vi "FlexMag process file.vi"() -> ()   [LabVIEW 2018]
panel:
  in  "process name":string
  out "count":dbl
  out "multiple":string
  out "single":string
  in  "SEARCH":bool
  in  "EXIT":bool
  in  "SAVE":bool
  in  "DELETE":bool
  in  "ADD":bool
  # "Process Name"
  # "Recipe Name"
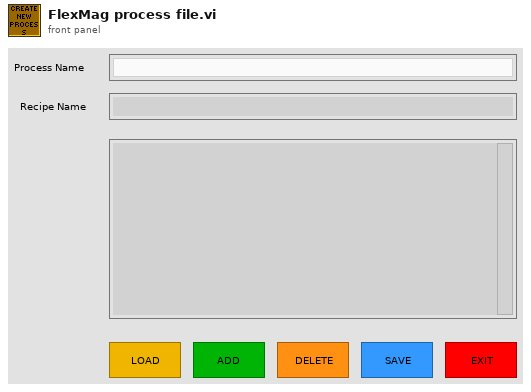
[diagram p1: front panel]
types:
  T1 = enum16{"open", "replace", "create", "open or create", "replace or create", "replace or create with confirmation"}
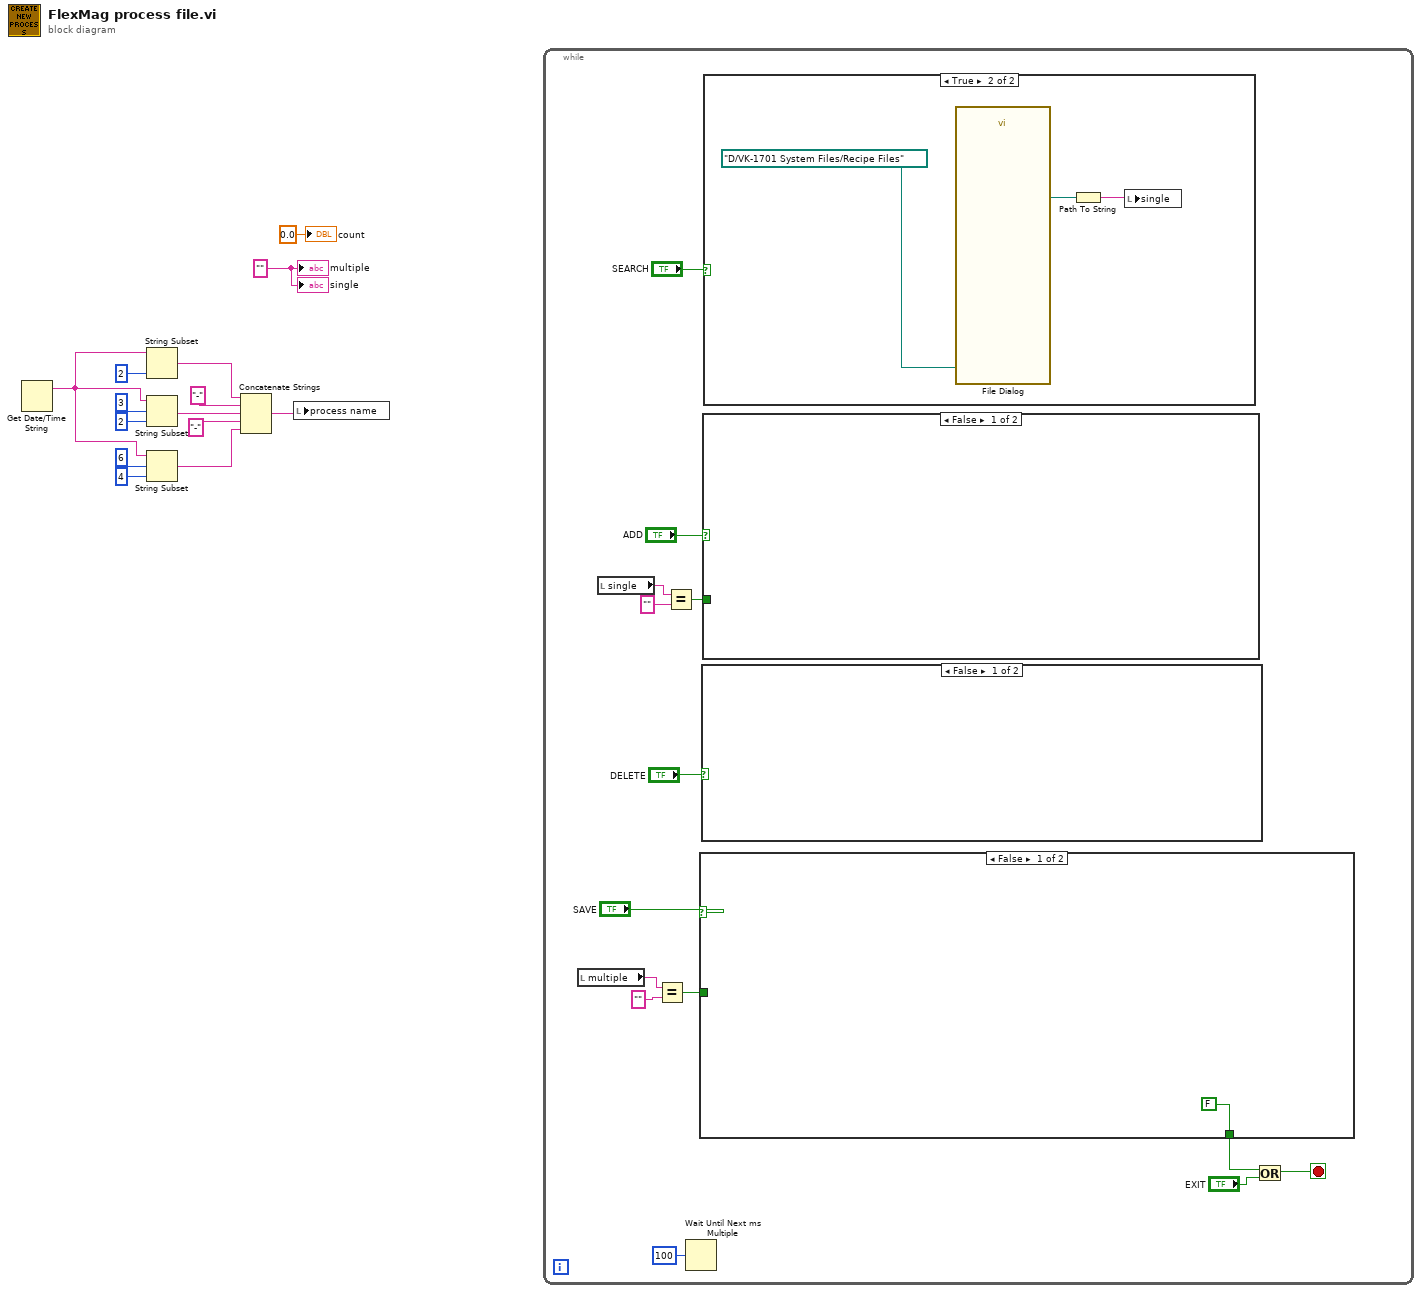
[diagram p0: block diagram]
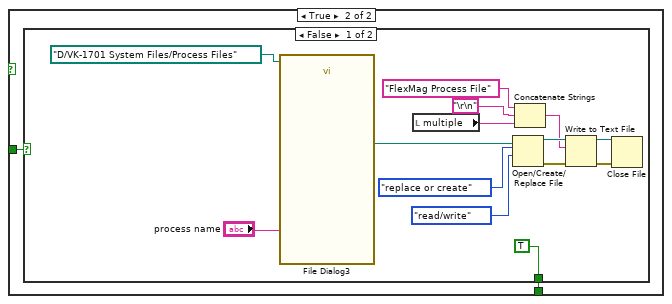
[diagram p3: hidden frame]
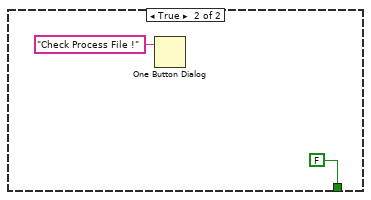
[diagram p4: hidden frame]
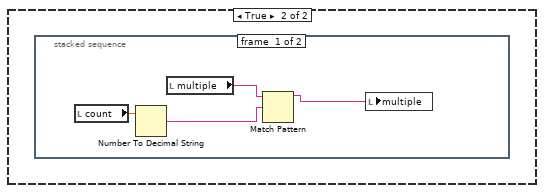
[diagram p5: hidden frame]
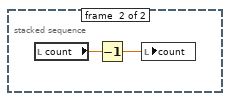
[diagram p6: hidden frame]
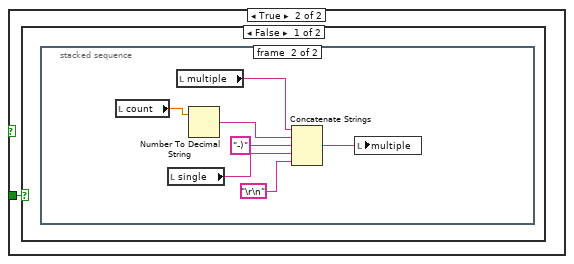
[diagram p7: hidden frame]
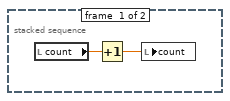
[diagram p8: hidden frame]
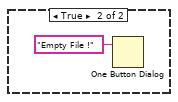
[diagram p9: hidden frame]
diagram:
  w13 = "" ("multiple")
  n1 = Get Date/Time String() -> (date string=w9:string)  [unwired: 3 in, 1 out]
  n2 = String Subset(string=w9, length (rest)=2 ("length (rest)")) -> (substring=w10:string)  [unwired: 1 in]
  n3 = String Subset(string=w9, offset (0)=3, length (rest)=2 ("length (rest)")) -> (substring=w11:string)
  n4 = String Subset(string=w9, offset (0)=6, length (rest)=4 ("length (rest)")) -> (substring=w12:string)
  n5 = Concatenate Strings(w10, "-" ("string"), w11, "-" ("string"), w12) -> (w1:string)
  n6 = local write "process name"(w1) -> ()
  n7 = while {
    stop <- w16 stop-if-true
    n8 = local read "multiple"() -> (w20:string)
    n9 = local read "single"() -> (w27:string)
    n10 = Equal?(x=w20, y="") -> (x = y?=w19:bool)
    n11 = Equal?(x=w27, y="") -> (x = y?=w25:bool)
    n12 = Wait Until Next ms Multiple(millisecond multiple=u32 100) -> ()  [unwired: 1 out]
    n13 = case shown="False" "SAVE" {
      tunnel: w19 -> [_ w34]
      tunnel: [FALSE w33] -> w17
      frame False {
      }
      frame True {
        n14 = case shown="False" w34 {
          tunnel: [TRUE FALSE] -> w33
          frame False {
            n15 = call "File Dialog3"("start path"=path "D:/VK-1701 System Files/Process Files", "default name"="process name") -> ("selected path"=w44:path)  [unwired: 10 in, 3 out]
            n16 = local read "multiple"() -> (w37:string)
            n17 = Open/Create/Replace File(file path (use dialog)=w44, operation (0:open)=T1."replace or create", access (0:read/write)=enum16{"read/write", "read-only", "write-only"}."read/write") -> (refnum out=w41:refnum<file>, error out=w40:errorcluster)  [unwired: 3 in, 1 out]
            n18 = Concatenate Strings("FlexMag Process File" ("y"), "\r\n", w37) -> (w38:string)
            n19 = Write to Text File(file (use dialog)=w41, text=w38, error in=w40) -> (refnum out=w43:refnum<file>, error out=w42:errorcluster)  [unwired: 1 in, 1 out]
            n20 = Close File(refnum=w43, error in=w42) -> ()  [unwired: 2 out]
          }
          frame True {
            n21 = One Button Dialog(message="Check Process File !") -> ()  [unwired: 1 in, 1 out]
          }
        }
      }
    }
    n22 = case shown="False" "DELETE" {
      frame False {
      }
      frame True {
        n23 = stacked-sequence {
          frame #0 {
            n24 = local read "count"() -> (w54:dbl)
            n25 = Number To Decimal String(number=w54) -> (decimal integer string=w52:string)  [unwired: 1 in]
            n26 = local read "multiple"() -> (w53:string)
            n27 = Match Pattern(string=w53, regular expression=w52) -> (before substring=w51:string)  [unwired: 1 in, 3 out]
            n28 = local write "multiple"(w51) -> ()
          }
          frame #1 {
            n29 = local read "count"() -> (w56:dbl)
            n30 = Decrement(x=w56) -> (x-1=w55:dbl)
            n31 = local write "count"(w55) -> ()
          }
        }
      }
    }
    n32 = case shown="False" "ADD" {
      tunnel: w25 -> [_ w57]
      frame False {
      }
      frame True {
        n33 = case shown="False" w57 {
          frame False {
            n34 = stacked-sequence {
              frame #0 {
                n35 = local read "count"() -> (w58:dbl)
                n36 = Increment(x=w58) -> (x+1=w59:dbl)
                n37 = local write "count"(w59) -> ()
              }
              frame #1 {
                n38 = local read "count"() -> (w66:dbl)
                n39 = local read "single"() -> (w63:string)
                n40 = local read "multiple"() -> (w61:string)
                n41 = Number To Decimal String(number=w66) -> (decimal integer string=w65:string)  [unwired: 1 in]
                n42 = Concatenate Strings(w61, w65, "-)" ("string"), w63, "\r\n") -> (w62:string)
                n43 = local write "multiple"(w62) -> ()
              }
            }
          }
          frame True {
            n44 = One Button Dialog(message="Empty File !") -> ()  [unwired: 1 in, 1 out]
          }
        }
      }
    }
    n45 = case shown="True" "SEARCH" {
      frame False {
      }
      frame True {
        n46 = call "File Dialog"("start path"=path "D:/VK-1701 System Files/Recipe Files") -> ("selected path"=w30:path)  [unwired: 11 in, 3 out]
        n47 = Path To String(path=w30) -> (string=w29:string)
        n48 = local write "single"(w29) -> ()
      }
    }
    n49 = Or(x=w17, y="EXIT") -> (x .or. y?=w16:bool)
  }
  "multiple" <- w13
  "count" <- 0.0 ("count")
  "single" <- w13
